vi "get_value.vi"(8 "error in (no error)":errorcluster, 10 "channel":dbl, 11 "Agilent 34980A in":refnum<class "Agilent 34980A.lvclass">) -> (0 "error out":errorcluster, 2 "value":string, 3 "Agilent 34980A out":refnum<class "Agilent 34980A.lvclass">)   [LabVIEW 2018, in "Agilent 34980A.lvclass"]
doc: "the vi reads the value (pressure, temp etc etc) from the instrument"
uses:
  Agilent 34980A.lvclass
  instrument.lvclass
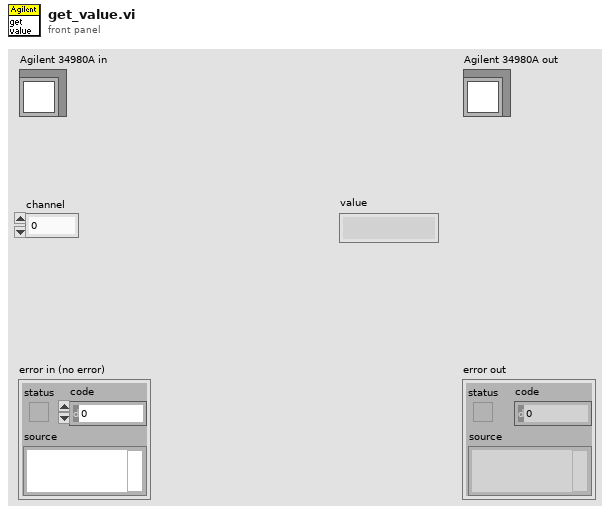
[diagram p1: front panel]
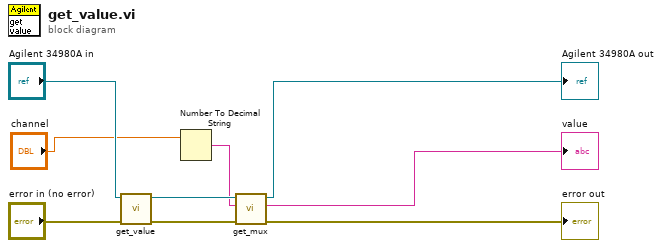
[diagram p0: block diagram]
diagram:
  n1 = call-parent "get_value.vi"("error in (no error)"="error in (no error)", "instrument in"="Agilent 34980A in") -> ("error out"=w6:errorcluster, "instrument out"=w7:refnum<class "Agilent 34980A.lvclass">)  [unwired: 7 in, 1 out]
  n2 = Number To Decimal String(number="channel") -> (decimal integer string=w3:string)  [unwired: 1 in]
  n3 = call-dynamic "get_mux.vi"("error in (no error)"=w6, "Channel"=w3, "Agilent 34980A in"=w7) -> ("error out"=→"error out":errorcluster, "value"=→"value":string, "Agilent 34980A out"=→"Agilent 34980A out":refnum<class "Agilent 34980A.lvclass">)  [unwired: 6 in]
